vi "ConfigStdWfrm.vi"(8 "error in (no error)":errorcluster, 11 "ClassIn":refnum<class "NiPxi6733.lvclass">) -> (0 "error out":errorcluster, 3 "ClassOut":refnum<class "NiPxi6733.lvclass">)   [LabVIEW 2014, in "FGenPlugins.lvlib" / "NiPxi6733.lvclass"]
uses:
  NiPxi6733.lvclass
  <vilib>/measure/NI_MABase.lvlib
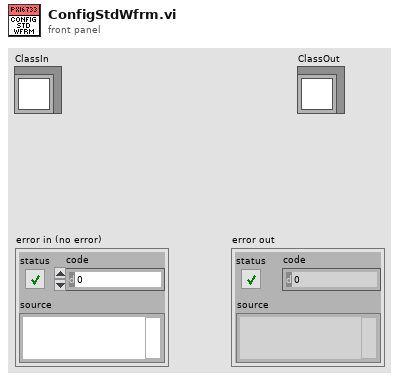
[diagram p1: front panel]
types:
  T1 = typedef "FGenPlugins.lvlib/NISTFGenPluginsBase.lvclass/StdWaveformParams.ctl" = cluster{"eWaveform":u16, "dAmplitude":dbl, "dDcOffset":dbl, "dFrequency":dbl, "dStartPhase":dbl, "dSampleRate":dbl, "dNumSamples":dbl}
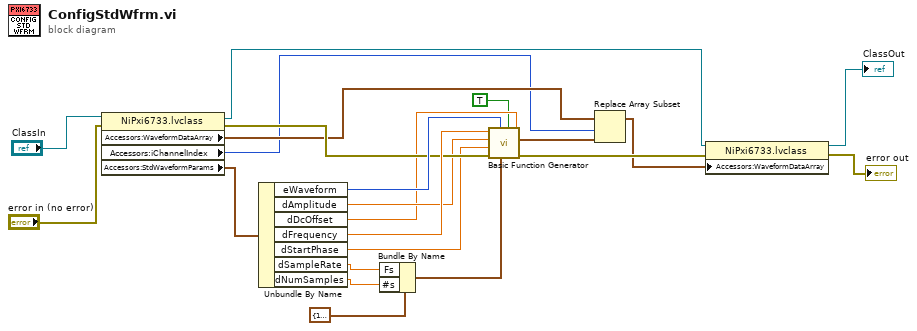
[diagram p0: block diagram]
diagram:
  n1 = property class="NiPxi6733.lvclass"(reference="ClassIn", error in="error in (no error)") -> (reference out=w11:refnum<class "NiPxi6733.lvclass">, error out=w16:errorcluster, "Accessors:WaveformDataArray"=w7:waveform(dbl)[], "Accessors:iChannelIndex"=w2:i32, "Accessors:StdWaveformParams"=w1:T1)
  n2 = Unbundle By Name(w1) -> ("eWaveform"=w18:u16, "dAmplitude"=w13:dbl, "dDcOffset"=w12:dbl, "dFrequency"=w17:dbl, "dStartPhase"=w14:dbl, "dSampleRate"=w5:dbl, "dNumSamples"=w4:dbl)
  n3 = Bundle By Name(cluster=cluster{"Fs":dbl, "#s":dbl} {"Fs"=1000.0, "#s"=1000.0} ("sampling info"), "Fs"=w5, "#s"=w4) -> (w3:cluster{"Fs":dbl, "#s":dbl})
  n4 = call <vilib>:"Basic Function Generator.vi"("offset"=w12, "reset signal"=TRUE, "sampling info"=w3, "signal type"=w18, "error in (no error)"=w16, "phase"=w14, "amplitude"=w13, "frequency"=w17) -> ("error out"=w15:errorcluster, "signal out"=w10:waveform(dbl))  [unwired: 1 in, 1 out]
  n5 = Replace Array Subset(array=w7, new element=w10, index=w2) -> (w8:waveform(dbl)[])
  n6 = property class="NiPxi6733.lvclass"(reference=w11, error in=w15, "Accessors:WaveformDataArray"=w8) -> (reference out=→"ClassOut":refnum<class "NiPxi6733.lvclass">, error out=→"error out":errorcluster)
